vi "LiDAR.vi"() -> ()   [LabVIEW 2020]
uses:
  47d84769-d6d3-4327-8500-e9d67ac4b2fd.vi
  612987ad-0ce6-4e08-b257-b00cf9bbbb63.vi
panel:
  out "Array 3":dbl[](array[numeric])
  out "array 3":dbl[](array[numeric])
  out "Array 2":dbl[](array[numeric])
  out "array 2":dbl[](array[numeric])
  out "size(s)":i32
  out "Y":i32
  out "X":i32
  out "array":dbl[](array[numeric])
  out "Mixed Signal Graph":cluster{dbl[], dbl[]}[](graph)
  in  "점 개수":i32
  in  "range(m)":dbl
  in  "channel 15":bool
  in  "channel 14":bool
  in  "channel 13":bool
  in  "channel 12":bool
  in  "channel 11":bool
  in  "channel 10":bool
  in  "channel 9":bool=TRUE
  in  "channel 8":bool=TRUE
  in  "channel 7":bool=TRUE
  in  "channel 6":bool=TRUE
  in  "channel 5":bool
  in  "channel 4":bool
  in  "channel 3":bool
  in  "channel 2":bool
  in  "channel 1":bool
  in  "channel 0":bool
  out "XY Graph":cluster{dbl[], dbl[]}(graph)
  out "seconds":dbl
  out "minutes":dbl
  out "Array":string[](array[string])
  out "TimeStamp & Factory":string
  out "Trans Array":string[](array[string])
  in  "stop":bool
  out "data out":string
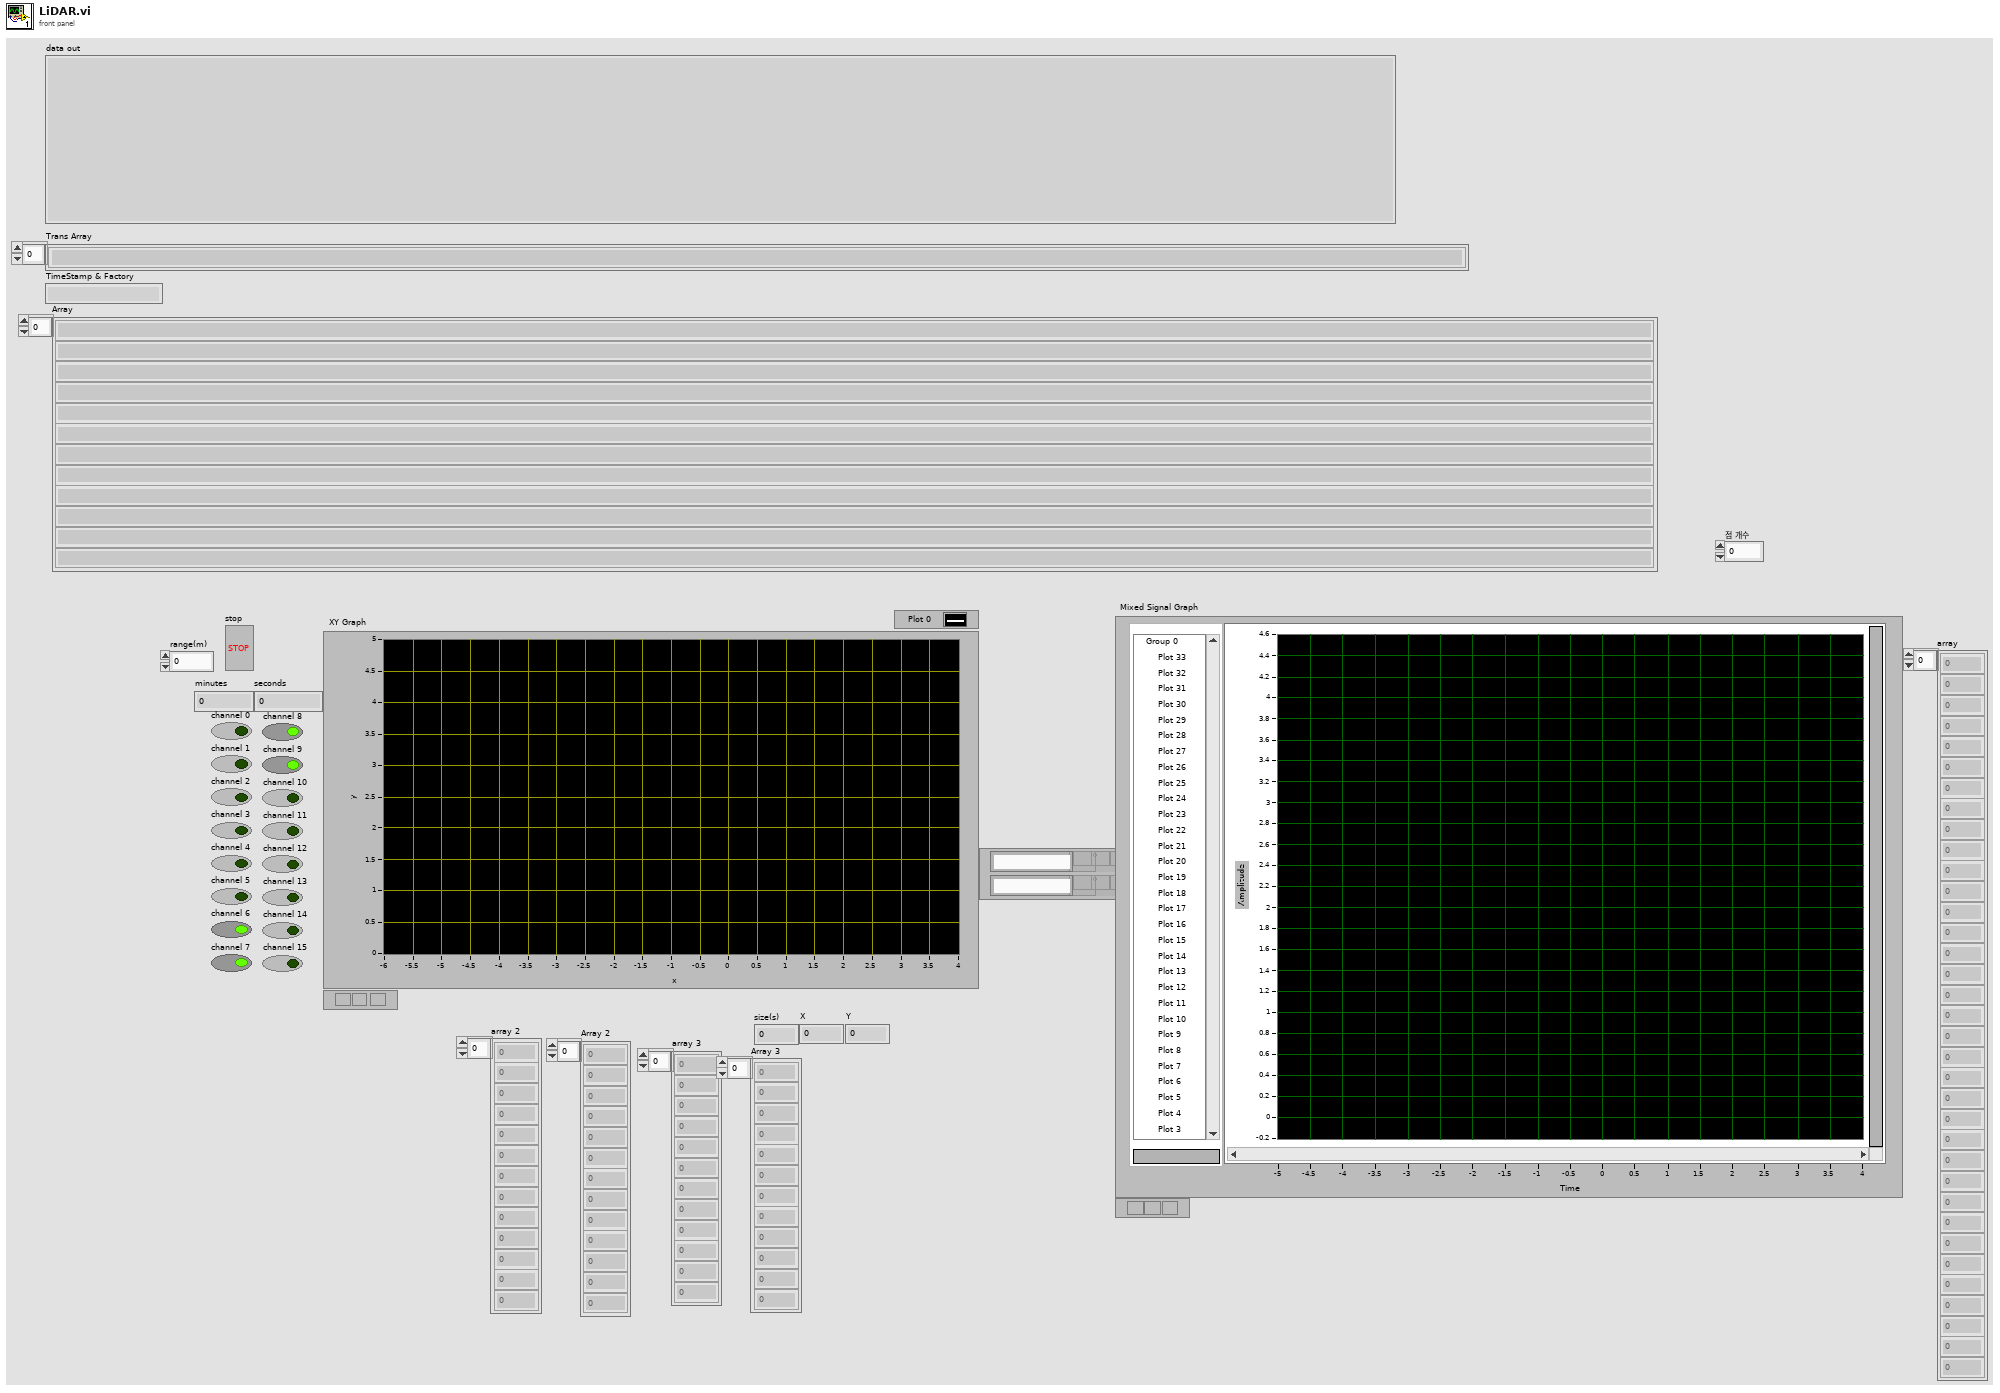
[diagram p1: front panel]
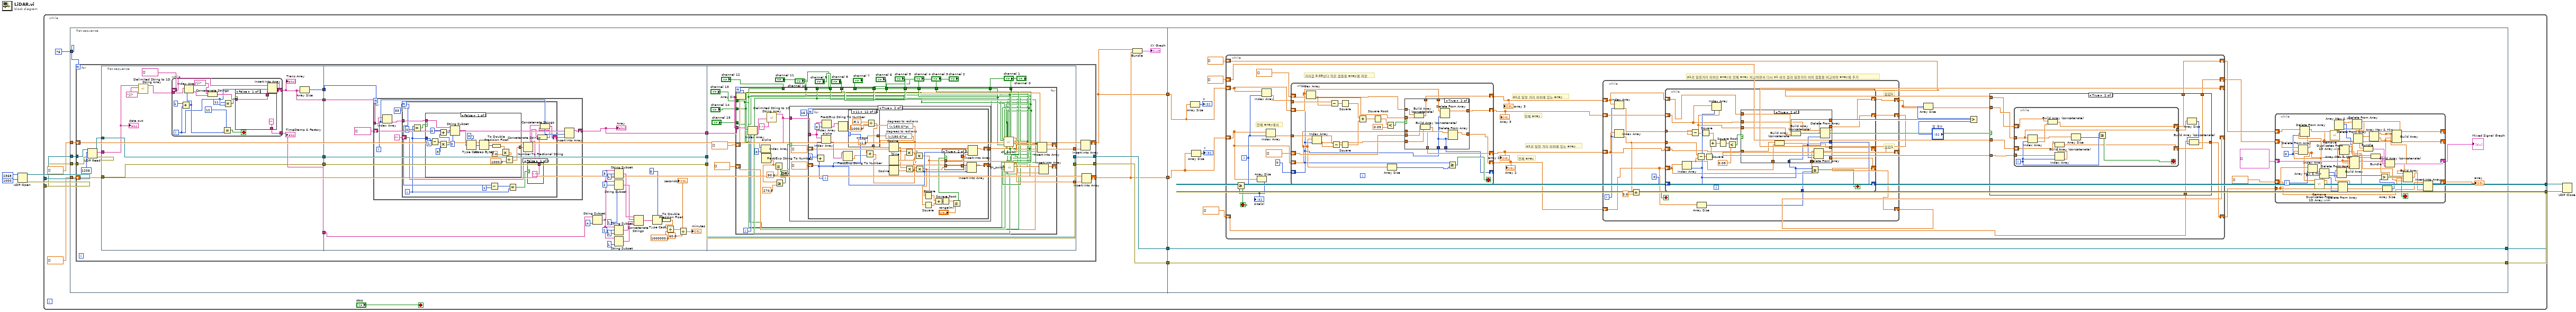
[diagram p0: block diagram]
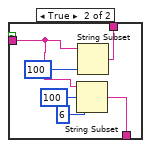
[diagram p2: hidden frame]
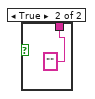
[diagram p3: hidden frame]
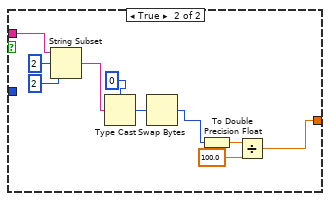
[diagram p4: hidden frame]
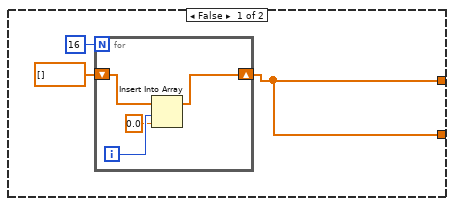
[diagram p5: hidden frame]
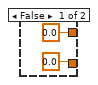
[diagram p6: hidden frame]
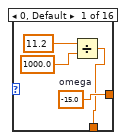
[diagram p7: hidden frame]
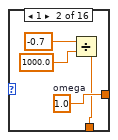
[diagram p8: hidden frame]
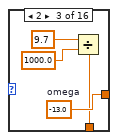
[diagram p9: hidden frame]
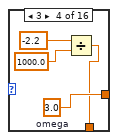
[diagram p10: hidden frame]
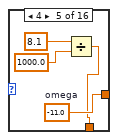
[diagram p11: hidden frame]
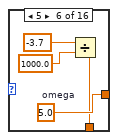
[diagram p12: hidden frame]
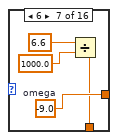
[diagram p13: hidden frame]
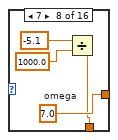
[diagram p14: hidden frame]
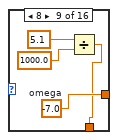
[diagram p15: hidden frame]
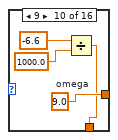
[diagram p16: hidden frame]
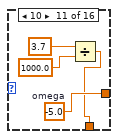
[diagram p17: hidden frame]
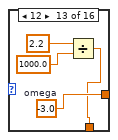
[diagram p18: hidden frame]
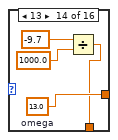
[diagram p19: hidden frame]
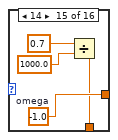
[diagram p20: hidden frame]
diagram:
  n1 = UDP Open(9:1000 ("timeout ms (25000)"), 11:u16 2368 ("port")) -> (port=w4:refnum<k16>, 0:w3:errorcluster)  [unwired: 3 in, 1 out]
  n2 = while {
    tunnel: w4 -> [w17]
    tunnel: w3 -> [w16]
    tunnel: [w12] -> w2
    tunnel: [w18] -> w1
    stop <- "stop" stop-if-true
    n3 = flat-sequence {
      tunnel: w17 -> [w27]
      tunnel: w16 -> [w26]
      tunnel: dbl[] [] -> [w25]
      tunnel: dbl[] [] -> [w24]
      tunnel: 76 -> [w22]
      tunnel: [w28] -> w10
      tunnel: [w23] -> w9
      tunnel: [w20] -> w8
      tunnel: [w19] -> w7
      tunnel: [w352] -> w12
      tunnel: [w353] -> w18
      tunnel: w10 -> [w353]
      tunnel: w9 -> [w352]
      tunnel: w8 -> [w345]
      tunnel: w7 -> [w344]
      frame #0 {
        n4 = for {
          N: w22 -> [_]
          tunnel: w27 -> [w39]
          tunnel: [w41] -> w23
          tunnel: w26 -> [w38]
          tunnel: [w42] -> w28
          shift-right: [w31] -> w19
          shift-left: w25 -> [w30]
          shift-right: [w33] -> w20
          shift-left: w24 -> [w29]
          n5 = UDP Read(connection ID=w39, max size (548)=1206, 8:w38) -> (data out=w35:string, error out=w36:errorcluster, 3:w37:refnum<k16>)  [unwired: 1 in, 2 out]
          n6 = flat-sequence {
            tunnel: [w53] -> w50
            tunnel: [w52] -> w49
            tunnel: [w56] -> w48
            tunnel: [w55] -> w47
            tunnel: [w54] -> w46
            tunnel: w36 -> [w53]
            tunnel: w37 -> [w52]
            tunnel: w35 -> [w51]
            tunnel: w50 -> [w110]
            tunnel: w49 -> [w109]
            tunnel: w48 -> [w108]
            tunnel: w47 -> [w107]
            tunnel: w46 -> [w105]
            tunnel: [w110] -> w45
            tunnel: [w109] -> w44
            tunnel: [w83] -> w43
            tunnel: [w185] -> w41
            tunnel: [w186] -> w42
            tunnel: w45 -> [w186]
            tunnel: w44 -> [w185]
            tunnel: w43 -> [w183]
            tunnel: [w180] -> w32
            tunnel: [w179] -> w34
            frame #0 {
              n7 = call <vilib>:"Delimited String to 1D String Array.vi"("delimiter"="ÿî", "delimited string"=w51) -> ("string array"=w57:string[])  [unwired: 9 in]
              n8 = while {
                tunnel: w57 -> [w74]
                shift-right: [w67] -> w55
                shift-left: string[] [] -> [w66]
                tunnel: [w60] -> w54
                i -> [w63]
                stop <- w68 stop-if-true
                n9 = Add(x=1, y=w63) -> (x+y=w70:i32)
                n10 = Index Array(array=w74, index=w70) -> (element=w73:string)
                n11 = Concatenate Strings("ÿî" ("delimiter"), w73) -> (w65:string)
                n12 = Equal?(x=12, y=w70) -> (x = y?=w68:bool)
                n13 = Equal?(x=11, y=w63) -> (x = y?=w61:bool)
                n14 = case shown="False" w61 {
                  tunnel: w65 -> [w76 w78]
                  tunnel: [w76 w81] -> w64
                  tunnel: ["" w77] -> w60
                  frame False {
                  }
                  frame True {
                    n15 = String Subset(string=w78, offset (0)=100, length (rest)=6 ("length (rest)")) -> (substring=w77:string)
                    n16 = String Subset(string=w78, length (rest)=100 ("length (rest)")) -> (substring=w81:string)  [unwired: 1 in]
                  }
                }
                n17 = Insert Into Array(array=w66, index=w63, new element=w64) -> (w67:string[])
              }
              "Trans Array" <- w55
              "TimeStamp & Factory" <- w54
              n18 = Array Size(array=w55) -> (size(s)=w56:i32)
              "data out" <- w51
            }
            frame #1 {
              n19 = for {
                N: w108 -> [_]
                tunnel: w107 -> [w118]
                shift-right: [w114] -> w83
                shift-left: string[] [] -> [w112]
                i -> [w115]
                n20 = Index Array(array=w118, index=w115) -> (element=w116:string)
                n21 = for {
                  N: 33 -> [w121]
                  tunnel: w116 -> [w130]
                  shift-right: [w123] -> w113
                  shift-left: "" -> [w122]
                  i -> [w129]
                  n22 = Equal?(x=w129, y=0) -> (x = y?=w131:bool)
                  n23 = case shown="False" w131 {
                    tunnel: w130 -> [w142 w160]
                    tunnel: w129 -> [w147 _]
                    tunnel: [w135 w153] -> w127
                    frame False {
                      n24 = Subtract(x=w147, y=1) -> (x-y=w148:i32)
                      n25 = Multiply(x=w148, y=3) -> (x*y=w144:i32)
                      n26 = Add(x=4 ("offset (0)"), y=w144) -> (x+y=w143:i32)
                      n27 = String Subset(string=w142, offset (0)=w143, length (rest)=2 ("length (rest)")) -> (substring=w141:string)
                      n28 = Type Cast(type=u16 0, x=w141) -> (*(type *) &x=w150:u16)
                      n29 = Swap Bytes(anything=w150) -> (byte swapped=w140:u16)
                      n30 = To Double Precision Float(number=w140) -> (double precision float=w139:dbl)
                      n31 = Multiply(x=w139, y=2.0) -> (x*y=w136:dbl)
                      n32 = Divide(x=w136, y=1000.0) -> (x/y=w135:dbl)
                    }
                    frame True {
                      n33 = String Subset(string=w160, offset (0)=2, length (rest)=2 ("length (rest)")) -> (substring=w157:string)
                      n34 = Type Cast(type=u16 0, x=w157) -> (*(type *) &x=w158:u16)
                      n35 = Swap Bytes(anything=w158) -> (byte swapped=w155:u16)
                      n36 = To Double Precision Float(number=w155) -> (double precision float=w156:dbl)
                      n37 = Divide(x=w156, y=100.0) -> (x/y=w153:dbl)
                    }
                  }
                  n38 = Subtract(x=w121, y=1) -> (x-y=w119:i32)
                  n39 = Equal?(x=w119, y=w129) -> (x = y?=w128:bool)
                  n40 = Number To Fractional String(number=w127) -> (F-format string=w126:string)  [unwired: 3 in]
                  n41 = case shown="False" w128 {
                    tunnel: ["," ""] -> w125
                    frame False {
                    }
                    frame True {
                    }
                  }
                  n42 = Concatenate Strings(w126, w125) -> (w124:string)
                  n43 = Concatenate Strings(w122, w124) -> (w123:string)
                }
                n44 = Insert Into Array(array=w112, index=w115, new element=w113) -> (w114:string[])
              }
              "Array" <- w83
              n45 = String Subset(string=w105, length (rest)=4 ("length (rest)")) -> (substring=w103:string)  [unwired: 1 in]
              n46 = String Subset(string=w103, offset (0)=3, length (rest)=1 ("length (rest)")) -> (substring=w95:string)
              n47 = String Subset(string=w103, offset (0)=2, length (rest)=1 ("length (rest)")) -> (substring=w94:string)
              n48 = String Subset(string=w103, offset (0)=1, length (rest)=1 ("length (rest)")) -> (substring=w93:string)
              n49 = String Subset(string=w103, length (rest)=1 ("length (rest)")) -> (substring=w92:string)  [unwired: 1 in]
              n50 = Concatenate Strings(w95, w94, w93, w92) -> (w90:string)
              n51 = Type Cast(type=u32 0, x=w90) -> (*(type *) &x=w89:u32)
              n52 = To Double Precision Float(number=w89) -> (double precision float=w88:dbl)
              n53 = Divide(x=w88, y=1000000.0) -> (x/y=w85:dbl)
              "seconds" <- w85
              n54 = Divide(x=w85, y=60.0) -> (x/y=→"minutes":dbl)
            }
            frame #2 {
              n55 = Array Size(array=w183) -> (size(s)=w184:i32)
              n56 = for {
                N: w184 -> [_]
                tunnel: w183 -> [w222]
                shift-right: [w219] -> w180
                shift-left: dbl[] [] -> [w218]
                shift-right: [w217] -> w179
                shift-left: dbl[] [] -> [w216]
                tunnel: "channel 0" -> [w211]
                tunnel: "channel 1" -> [w210]
                tunnel: "channel 2" -> [w209]
                tunnel: "channel 3" -> [w208]
                tunnel: "channel 4" -> [w207]
                tunnel: "channel 5" -> [w206]
                tunnel: "channel 6" -> [w205]
                tunnel: "channel 7" -> [w204]
                tunnel: "channel 8" -> [w203]
                tunnel: "channel 9" -> [w202]
                tunnel: "channel 10" -> [w201]
                tunnel: "channel 11" -> [w200]
                tunnel: "channel 12" -> [w199]
                tunnel: "channel 13" -> [w198]
                tunnel: "channel 14" -> [w197]
                tunnel: "channel 15" -> [w196]
                i -> [w220]
                n57 = Index Array(array=w222, index=w220) -> (element=w221:string)
                n58 = call <vilib>:"Delimited String to 1D String Array.vi"("delimiter"=",", "delimited string"=w221) -> ("string array"=w195:string[])  [unwired: 9 in]
                n59 = Index Array "alpha"(array=w195, index=0) -> (element=w193:string)
                n60 = Fract/Exp String To Number(string=w193) -> (number=w191:dbl)  [unwired: 3 in, 1 out]
                n61 = Less Or Equal?(x=w191, y=90.0 ("작거나같다")) -> (x <= y?=w189:bool)
                n62 = Greater Or Equal?(x=w191, y=270.0 ("크거나같다")) -> (x >= y?=w188:bool)
                n63 = Or(x=w189, y=w188) -> (x .or. y?=w187:bool)
                n64 = case shown="True" w187 {
                  tunnel: [w224 w233] -> w213
                  tunnel: [w224 w232] -> w212
                  tunnel: w195 -> [_ w231]
                  frame False {
                    n65 = for {
                      N: 16 -> [_]
                      shift-right: [w230] -> w224
                      shift-left: dbl[] [] -> [w227]
                      i -> [w229]
                      n66 = Insert Into Array(array=w227, index=w229, new element=0.0 ("new element/subarray")) -> (w230:dbl[])
                    }
                  }
                  frame True {
                    n67 = for {
                      N: 16 -> [_]
                      tunnel: w231 -> [w267]
                      shift-right: [w254] -> w233
                      shift-left: dbl[] [] -> [w253]
                      shift-right: [w251] -> w232
                      shift-left: dbl[] [] -> [w250]
                      i -> [w252]
                      n68 = Add(x=1, y=w252) -> (x+y=w268:i32)
                      n69 = Index Array(array=w267, index=w268) -> (element=w264:string)
                      n70 = Index Array "alpha"(array=w267, index=0) -> (element=w265:string)
                      n71 = Fract/Exp String To Number(string=w265) -> (number=w255:dbl)  [unwired: 3 in, 1 out]
                      n72 = Fract/Exp String To Number(string=w264) -> (number=w248:dbl)  [unwired: 3 in, 1 out]
                      n73 = case shown="11" w252 {
                        tunnel: [w277 w281 w285 w289 w293 w297 w301 w305 w309 w313 w317 w321 w325 w329 w333 w337] -> w263
                        tunnel: [w274 w278 w282 w286 w290 w294 w298 w302 w306 w310 w314 w318 w322 w326 w330 w334] -> w249
                        frame 0, Default {
                          w277 = -15.0  # omega
                          n74 = Divide(x=11.2, y=1000.0) -> (x/y=w274:dbl)
                        }
                        frame 1 {
                          w281 = 1.0  # omega
                          n75 = Divide(x=-0.7, y=1000.0) -> (x/y=w278:dbl)
                        }
                        frame 2 {
                          w285 = -13.0  # omega
                          n76 = Divide(x=9.7, y=1000.0) -> (x/y=w282:dbl)
                        }
                        frame 3 {
                          w289 = 3.0  # omega
                          n77 = Divide(x=-2.2, y=1000.0) -> (x/y=w286:dbl)
                        }
                        frame 4 {
                          w293 = -11.0  # omega
                          n78 = Divide(x=8.1, y=1000.0) -> (x/y=w290:dbl)
                        }
                        frame 5 {
                          w297 = 5.0  # omega
                          n79 = Divide(x=-3.7, y=1000.0) -> (x/y=w294:dbl)
                        }
                        frame 6 {
                          w301 = -9.0  # omega
                          n80 = Divide(x=6.6, y=1000.0) -> (x/y=w298:dbl)
                        }
                        frame 7 {
                          w305 = 7.0  # omega
                          n81 = Divide(x=-5.1, y=1000.0) -> (x/y=w302:dbl)
                        }
                        frame 8 {
                          w309 = -7.0  # omega
                          n82 = Divide(x=5.1, y=1000.0) -> (x/y=w306:dbl)
                        }
                        frame 9 {
                          w313 = 9.0  # omega
                          n83 = Divide(x=-6.6, y=1000.0) -> (x/y=w310:dbl)
                        }
                        frame 10 {
                          w317 = -5.0  # omega
                          n84 = Divide(x=3.7, y=1000.0) -> (x/y=w314:dbl)
                        }
                        frame 11 {
                          w321 = 11.0  # omega
                          n85 = Divide(x=-8.1, y=1000.0) -> (x/y=w318:dbl)
                        }
                        frame 12 {
                          w325 = -3.0  # omega
                          n86 = Divide(x=2.2, y=1000.0) -> (x/y=w322:dbl)
                        }
                        frame 13 {
                          w329 = 13.0  # omega
                          n87 = Divide(x=-9.7, y=1000.0) -> (x/y=w326:dbl)
                        }
                        frame 14 {
                          w333 = -1.0  # omega
                          n88 = Divide(x=0.7, y=1000.0) -> (x/y=w330:dbl)
                        }
                        frame 15 {
                          w337 = 15.0  # omega
                          n89 = Divide(x=-11.2, y=1000.0) -> (x/y=w334:dbl)
                        }
                      }
                      n90 = Add(x=w249, y=w248) -> (x+y=w247:dbl)
                      n91 = expression code="(x/180.0)*pi" "degrees to radians"(w263) -> (w262:dbl)
                      n92 = expression code="(x/180.0)*pi" "degrees to radians"(w255) -> (w261:dbl)
                      n93 = Cosine(x=w262) -> (cos(x)=w259:dbl)
                      n94 = Sine(x=w261) -> (sin(x)=w260:dbl)
                      n95 = Cosine(x=w261) -> (cos(x)=w258:dbl)
                      n96 = Multiply(x=w259, y=w260) -> (x*y=w256:dbl)
                      n97 = Multiply(x=w259, y=w258) -> (x*y=w257:dbl)
                      n98 = Multiply "x"(x=w256, y=w247) -> (x*y=w241:dbl)
                      n99 = Multiply "y"(x=w257, y=w247) -> (x*y=w239:dbl)
                      n100 = Square(x=w241) -> (x^2=w246:dbl)
                      n101 = Square(x=w239) -> (x^2=w245:dbl)
                      n102 = Add(x=w246, y=w245) -> (x+y=w244:dbl)
                      n103 = Square Root(x=w244) -> (sqrt(x)=w243:dbl)
                      n104 = Less Or Equal?(x=w243, y="range(m)") -> (x <= y?=w242:bool)
                      n105 = case shown="True" w242 {
                        tunnel: w241 -> [_ w273]
                        tunnel: [0.0 w273] -> w240
                        tunnel: w239 -> [_ w272]
                        tunnel: [0.0 w272] -> w238
                        frame False {
                        }
                        frame True {
                        }
                      }
                      n106 = Insert Into Array(array=w250, index=w252, new element=w238) -> (w251:dbl[])
                      n107 = Insert Into Array(array=w253, index=w252, new element=w240) -> (w254:dbl[])
                    }
                  }
                }
                n108 = call "ch_switch.vi"("channel 14"=w197, "channel 4"=w207, "channel 13"=w198, "channel 5"=w206, "channel 12"=w199, "channel 6"=w205, "channel 7"=w204, "channel 3"=w208, "channel 8"=w203, "channel 15"=w196, "channel 9"=w202, "channel 2"=w209, "channel 10"=w201, "channel 1"=w210, "channel 11"=w200, "channel 0"=w211, "Array in"=w213) -> ("Array out"=w214:dbl[])  [unwired: 10 in]
                n109 = call "ch_switch.vi"("channel 14"=w197, "channel 4"=w207, "channel 13"=w198, "channel 5"=w206, "channel 12"=w199, "channel 6"=w205, "channel 7"=w204, "channel 3"=w208, "channel 8"=w203, "channel 15"=w196, "channel 9"=w202, "channel 2"=w209, "channel 10"=w201, "channel 1"=w210, "channel 11"=w200, "channel 0"=w211, "Array in"=w212) -> ("Array out"=w215:dbl[])  [unwired: 10 in]
                n110 = Insert Into Array(array=w218, new element=w214) -> (w219:dbl[])  [unwired: 1 in]
                n111 = Insert Into Array(array=w216, new element=w215) -> (w217:dbl[])  [unwired: 1 in]
              }
            }
          }
          n112 = Insert Into Array(array=w30, new element=w32) -> (w31:dbl[])  [unwired: 1 in]
          n113 = Insert Into Array(array=w29, new element=w34) -> (w33:dbl[])  [unwired: 1 in]
        }
        n114 = Bundle(w19, w20) -> (→"XY Graph":cluster{dbl[], dbl[]})  [unwired: 1 in]
      }
      frame #1 {
        n115 = Array Size(array=w344) -> (size(s)=→"X":i32)
        n116 = Array Size(array=w345) -> (size(s)=→"Y":i32)
        n117 = while {
          shift-right: [w396] -> _
          shift-left: w344 -> [w405]
          shift-right: [w400] -> _
          shift-left: w345 -> [w404]
          shift-right: [w397] -> w348
          shift-left: dbl[] [] -> [w399]
          shift-right: [w394] -> w347
          shift-left: dbl[] [] -> [w398]
          shift-right: [w392] -> w346
          shift-left: dbl[] [] -> [w393]
          i -> [w413]
          stop <- w414 stop-if-true
          # "전체 array에서"
          # "전체 array"
          # "p1과 일정 거리 이하에 있는 array"
          # "전체 array"
          # "p1과 일정거리 이하인 array와 전체 array 비교하면서 다시 p1 외의 점과 일정거리 이하 점들을 비교하며 array에 추가"
          # "p1과 일정 거리 이하에 있는 array"
          # "거리값 0.05보다 작은 점들을 array에 저장"
          n118 = Array Size(array=w404) -> (size(s)=w415:i32)
          "size(s)" <- w415
          n119 = Greater Or Equal?(x=w413, y=w415) -> (x >= y?=w414:bool)
          n120 = Index Array(array=w405, index=w413) -> (element=w412:dbl)
          n121 = Index Array(array=w404, index=w413) -> (element=w411:dbl)
          n122 = while {
            tunnel: w412 -> [w520]
            tunnel: w411 -> [w519]
            shift-right: [w505] -> w395
            shift-left: dbl[] [] ("array") -> [w507]
            shift-right: [w506] -> w391
            shift-left: dbl[] [] ("array") -> [w508]
            shift-right: [w502] -> w390
            shift-left: w405 -> [w504]
            shift-right: [w501] -> w389
            shift-left: w404 -> [w503]
            shift-right: [w497] -> _
            shift-left: 0 -> [w498]
            stop <- w499 stop-if-true
            n123 = Index Array(array=w504, index=w498) -> (element=w510:dbl)
            n124 = Index Array(array=w503, index=w498) -> (element=w509:dbl)
            n125 = Subtract(x=w520, y=w510) -> (x-y=w518:dbl)
            n126 = Subtract(x=w519, y=w509) -> (x-y=w517:dbl)
            n127 = Square(x=w517) -> (x^2=w515:dbl)
            n128 = Square(x=w518) -> (x^2=w516:dbl)
            n129 = Add(x=w516, y=w515) -> (x+y=w514:dbl)
            n130 = Square Root(x=w514) -> (sqrt(x)=w513:dbl)
            n131 = Less?(x=w513, y=0.09) -> (x < y?=w511:bool)
            n132 = Array Size(array=w503) -> (size(s)=w500:i32)
            n133 = case shown="True" w511 {
              tunnel: w508 -> [w527 w535]
              tunnel: w507 -> [w526 w532]
              tunnel: w510 -> [_ w534]
              tunnel: w509 -> [_ w531]
              tunnel: [w527 w533] -> w506
              tunnel: [w526 w530] -> w505
              tunnel: w504 -> [w525 w538]
              tunnel: [w525 w529] -> w502
              tunnel: w503 -> [w524 w537]
              tunnel: [w524 w536] -> w501
              tunnel: w498 -> [w522 w528]
              tunnel: [w521 w528] -> w497
              frame False {
                n134 = Add(x=1, y=w522) -> (x+y=w521:i32)
              }
              frame True {
                n135 = Build Array (concatenate)(w535, w534) -> (w533:dbl[])
                n136 = Build Array (concatenate)(w532, w531) -> (w530:dbl[])
                n137 = Delete From Array(array=w538, index=w528) -> (array with subset deleted=w529:dbl[])  [unwired: 1 in, 1 out]
                n138 = Delete From Array(array=w537, index=w528) -> (array with subset deleted=w536:dbl[])  [unwired: 1 in, 1 out]
              }
            }
            n139 = Greater Or Equal?(x=w498, y=w500) -> (x >= y?=w499:bool)
          }
          "array 2" <- w395
          "Array 2" <- w389
          "array 3" <- w391
          "Array 3" <- w390
          n140 = while {
            shift-right: [w446] -> w402
            shift-left: w391 -> [w449]
            shift-right: [w452] -> w401
            shift-left: w395 -> [w451]
            shift-right: [w447] -> w396
            shift-left: w390 -> [w450]
            shift-right: [w453] -> w400
            shift-left: w389 -> [w440]
            i -> [w445]
            stop <- w442 stop-if-true
            # "집합1"
            # "집합1"
            n141 = Index Array(array=w451, index=w445) -> (element=w443:dbl)
            n142 = Index Array(array=w449, index=w445) -> (element=w448:dbl)
            n143 = Equal?(x=w443, y=0.0) -> (x = y?=w442:bool)
            n144 = Array Size(array=w440) -> (size(s)=w441:i32)
            n145 = while {
              tunnel: w448 -> [w478]
              tunnel: w443 -> [w477]
              shift-right: [w465] -> _
              shift-left: 0 -> [w466]
              shift-right: [w461] -> w452
              shift-left: w451 -> [w458]
              shift-right: [w457] -> w446
              shift-left: w449 -> [w464]
              shift-right: [w456] -> w447
              shift-left: w450 -> [w460]
              shift-right: [w463] -> w453
              shift-left: w440 -> [w462]
              tunnel: w441 -> [w455]
              stop <- w467 stop-if-true
              n146 = Index Array(array=w462, index=w466) -> (element=w459:dbl)
              n147 = Subtract(x=w477, y=w459) -> (x-y=w475:dbl)
              n148 = Square(x=w475) -> (x^2=w474:dbl)
              n149 = Index Array(array=w460, index=w466) -> (element=w468:dbl)
              n150 = Subtract(x=w478, y=w468) -> (x-y=w476:dbl)
              n151 = Square(x=w476) -> (x^2=w473:dbl)
              n152 = Add(x=w473, y=w474) -> (x+y=w472:dbl)
              n153 = Square Root(x=w472) -> (sqrt(x)=w471:dbl)
              n154 = Less?(x=w471, y=0.09) -> (x < y?=w469:bool)
              n155 = case shown="True" w469 {
                tunnel: w460 -> [w479 w488]
                tunnel: w466 -> [w484 w493]
                tunnel: w468 -> [_ w496]
                tunnel: [w480 w486] -> w457
                tunnel: w458 -> [w482 w495]
                tunnel: w464 -> [w480 w489]
                tunnel: w462 -> [w485 w494]
                tunnel: [w479 w490] -> w456
                tunnel: [w485 w491] -> w463
                tunnel: [w483 w493] -> w465
                tunnel: [w482 w492] -> w461
                tunnel: w459 -> [_ w487]
                frame False {
                  n156 = Add(x=1, y=w484) -> (x+y=w483:i32)
                }
                frame True {
                  n157 = Build Array (concatenate)(w495, w487) -> (w492:dbl[])
                  n158 = Build Array (concatenate)(w489, w496) -> (w486:dbl[])
                  n159 = Delete From Array(array=w494, index=w493) -> (array with subset deleted=w491:dbl[])  [unwired: 1 in, 1 out]
                  n160 = Delete From Array(array=w488, index=w493) -> (array with subset deleted=w490:dbl[])  [unwired: 1 in, 1 out]
                }
              }
              n161 = Greater Or Equal?(x=w466, y=w455) -> (x >= y?=w467:bool)
            }
          }
          n162 = Array Size(array=w402) -> (size(s)=w407:i32)
          n163 = Greater?(x=w407, y="점 개수") -> (0:w408:bool)
          n164 = case shown="True" w408 {
            tunnel: w402 -> [_ w428]
            tunnel: w401 -> [_ w427]
            tunnel: w399 -> [w418 w426]
            tunnel: w398 -> [w417 w425]
            tunnel: [w418 w422] -> w397
            tunnel: [w417 w424] -> w394
            tunnel: w393 -> [w416 w421]
            tunnel: [w416 w420] -> w392
            frame False {
            }
            frame True {
              n165 = while {
                shift-right: [w431] -> w422
                shift-left: w426 -> [w434]
                tunnel: w428 -> [w429]
                shift-right: [w430] -> w424
                shift-left: w425 -> [w433]
                tunnel: w427 -> [w439]
                tunnel: [w429] -> w419
                i -> [w438]
                stop <- w436 stop-if-true
                n166 = Index Array(array=w429, index=w438) -> (element=w435:dbl)
                n167 = Build Array (concatenate)(w434, w435) -> (w431:dbl[])
                n168 = Index Array(array=w439, index=w438) -> (element=w432:dbl)
                n169 = Build Array (concatenate)(w433, w432) -> (w430:dbl[])
                n170 = Array Size(array=w429) -> (size(s)=w437:i32)
                n171 = Greater Or Equal?(x=w438, y=w437) -> (x >= y?=w436:bool)
              }
              n172 = Array Size(array=w419) -> (size(s)=w423:i32)
              n173 = Build Array (concatenate)(w421, w423) -> (w420:dbl[])
            }
          }
        }
        n174 = while {
          shift-right: [w383] -> _
          shift-left: w348 -> [w388]
          shift-right: [w380] -> _
          shift-left: w347 -> [w381]
          tunnel: w346 -> [w384]
          shift-right: [w378] -> w338
          shift-left: cluster{dbl[], dbl[]}[] [] -> [w377]
          shift-right: [w354] -> w339
          shift-left: dbl[] [] ("array") -> [w356]
          i -> [w385]
          stop <- w386 stop-if-true
          w376 = 0 ("index")
          n175 = Index Array(array=w384, index=w385) -> (element=w382:dbl)
          n176 = Delete From Array(array=w381, length=w382, index=w376) -> (deleted portion=w367:dbl[], array with subset deleted=w380:dbl[])
          n177 = Delete From Array(array=w388, length=w382, index=w376) -> (deleted portion=w373:dbl[], array with subset deleted=w383:dbl[])
          n178 = call "Remove Duplicates From 1D Array.vim"("array"=w367) -> ("array with duplicates removed"=w365:dbl[])  [unwired: 10 in]
          n179 = Array Max & Min(array=w365) -> (max index (indices)=w363:i32, min index (indices)=w366:i32)  [unwired: 2 out]
          n180 = call "Remove Duplicates From 1D Array.vim"("array"=w373) -> ("array with duplicates removed"=w371:dbl[])  [unwired: 10 in]
          n181 = Array Max & Min(array=w371) -> (max index (indices)=w370:i32, min index (indices)=w372:i32)  [unwired: 2 out]
          n182 = Delete From Array(array=w365, index=w366) -> (array with subset deleted=w364:dbl[])  [unwired: 1 in, 1 out]
          n183 = Delete From Array(array=w364, index=w363) -> (array with subset deleted=w362:dbl[])  [unwired: 1 in, 1 out]
          n184 = Array Max & Min(array=w362) -> (max value=w358:dbl, min value=w357:dbl)  [unwired: 2 out]
          n185 = Build Array(w358, w357, w357, w358, w358) -> (w375:dbl[])
          n186 = Delete From Array(array=w371, index=w372) -> (array with subset deleted=w369:dbl[])  [unwired: 1 in, 1 out]
          n187 = Delete From Array(array=w369, index=w370) -> (array with subset deleted=w368:dbl[])  [unwired: 1 in, 1 out]
          n188 = Array Max & Min(array=w368) -> (max value=w360:dbl, min value=w359:dbl)  [unwired: 2 out]
          n189 = Bundle(w373, w367) -> (w379:cluster{dbl[], dbl[]})  [unwired: 1 in]
          n190 = Array Size(array=w384) -> (size(s)=w387:i32)
          n191 = Greater?(x=w385, y=w387) -> (0:w386:bool)
          n192 = Build Array(w360, w360, w359, w359, w360) -> (w374:dbl[])
          n193 = Bundle(w374, w375) -> (w361:cluster{dbl[], dbl[]})  [unwired: 1 in]
          n194 = Build Array (concatenate)(w377, w379, w361) -> (w378:cluster{dbl[], dbl[]}[])
          n195 = Build Array(w360, w359, w358, w357) -> (w355:dbl[])
          n196 = Insert Into Array(array=w356, new element=w355) -> (w354:dbl[])  [unwired: 1 in]
        }
        "array" <- w339
        "Mixed Signal Graph" <- w338
      }
    }
  }
  n197 = UDP Close(connection ID=w2, 8:w1) -> ()  [unwired: 2 out]
